vi "AIT 1553 - ReadWrite Message.vi"(5 "Mode":T9, 7 "Iteration":i32, 8 "error in (no error)":errorcluster, 9 "Bus Section":T1, 10 "FIFOs In":T2, 11 "Message In":T3 {"Driver Data"."First Word" min=8 max=31; "Driver Data"."Num Bits" min=1 max=32; "Driver Data"."Start Bit" min=8 max=31; "Block Data Refs"."Data Reference" format="%.0x"}) -> (0 "error out":errorcluster, 2 "FIFOs Out":T2, 3 "Message Out":T3 {"Driver Data"."First Word" min=8 max=31; "Driver Data"."Num Bits" min=1 max=32; "Driver Data"."Start Bit" min=8 max=31; "Block Data Refs"."Data Reference" format="%.0x"})   [LabVIEW 2014, in "AIT 1553 Custom Device.lvlib"]
uses:
  AIT 1553 Custom Device.lvlib
  RT Controls/ReadWrite Selector.ctl
  RT Controls/AIT 1553 - RT Message Settings.ctl
  <vilib>/NI Veristand/Custom Device API/Block Data Reference.ctl
  <vilib>/NI Veristand/Custom Device API/Data Reference.ctl
  RT Controls/AIT 1553 - Driver Data.ctl
  Controls and Global/Start Bit.ctl
  Controls and Global/Number of Bits.ctl
  RT Controls/FIFO.ctl
  RT Controls/AIT 1553 - Bus Section.ctl
  <vilib>/NI Veristand/Custom Device API/Global Data Refs.vi
  <vilib>/NI Veristand/Custom Device API/Custom Device API.lvlib
  <vilib>/NI Veristand/Custom Device Tools/Custom Device Utility Library/Custom Device Utility Library.lvlib
  <vilib>/NI Veristand/Custom Device Tools/Custom Device Utility Library/RT Debug String Color Spec.ctl
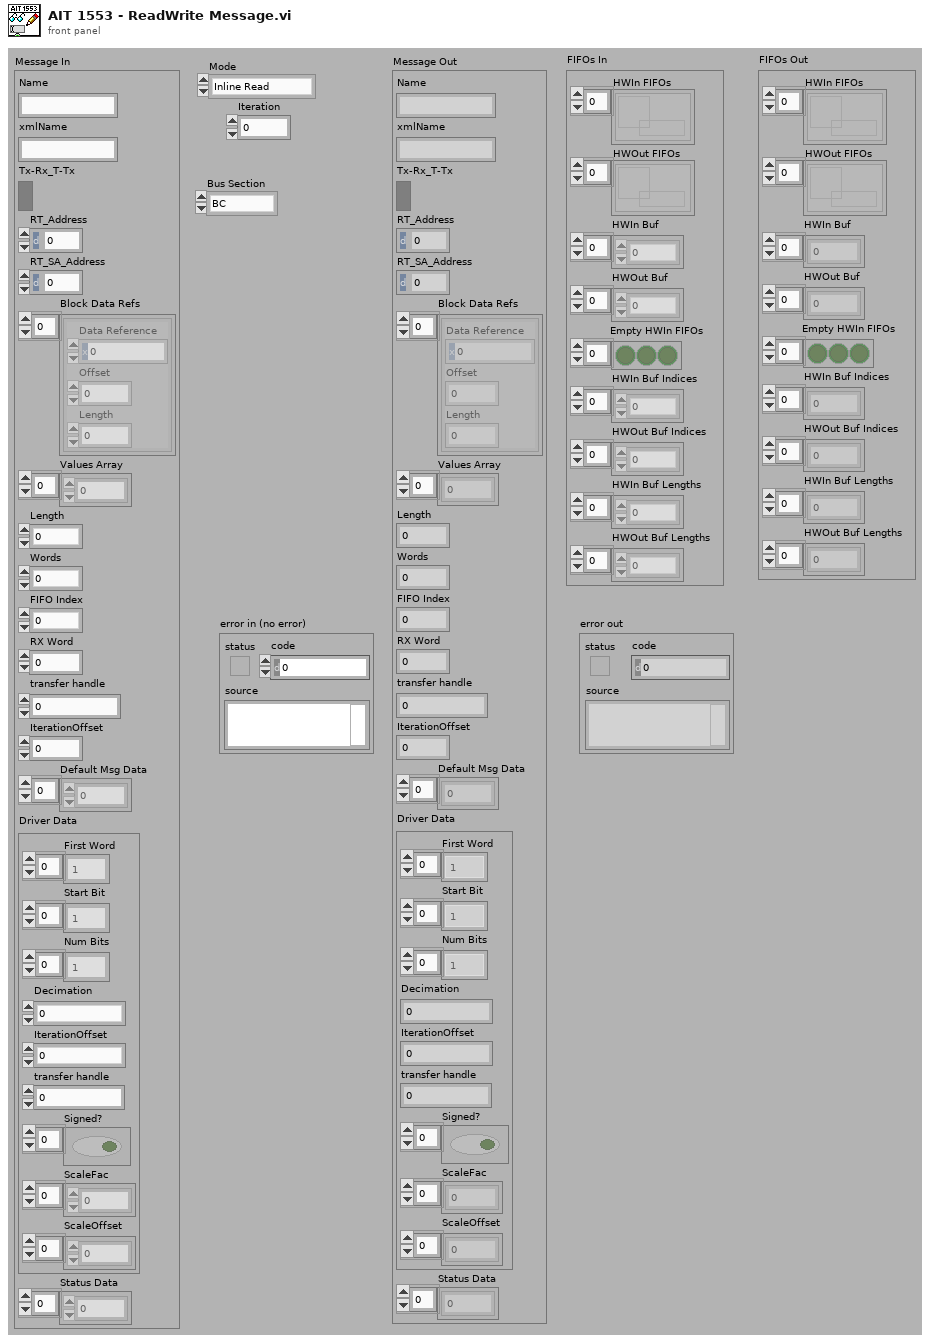
[diagram p1: front panel]
types:
  T1 = typedef "AIT 1553 Custom Device.lvlib/AIT 1553 - Bus Section.ctl" = enum16{"BC", "BM", "RT"}
  T2 = typedef "AIT 1553 Custom Device.lvlib/FIFO.ctl" = cluster{"HWIn FIFOs":refnum<k33>[], "HWOut FIFOs":refnum<k33>[], "HWIn Buf":dbl[], "HWOut Buf":dbl[], "Empty HWIn FIFOs":bool[], "HWIn Buf Indices":i32[], "HWOut Buf Indices":i32[], "HWIn Buf Lengths":i32[], "HWOut Buf Lengths":i32[]}
  T3 = typedef "AIT 1553 Custom Device.lvlib/AIT 1553 - RT Message Settings.ctl" = cluster{"Name":string, "xmlName":string, "Tx-Rx_T-Tx":bool, "RT_Address":u8, "RT_SA_Address":u8, "Block Data Refs":T4[], "Values Array":dbl[], "Length":i32, "Words":i32, "FIFO Index":i32, "RX Word":u32, "transfer handle":u32, "IterationOffset":i32, "Default Msg Data":u16[], "Driver Data":T6, "Status Data":u32[]}
  T4 = typedef "Custom Device API.lvlib/Block Data Reference.ctl" = cluster{"Data Reference":T5, "Offset":i32, "Length":i32}
  T5 = typedef "Custom Device API.lvlib/Data Reference.ctl" = i32
  T6 = typedef "AIT 1553 Custom Device.lvlib/AIT 1553 - Driver Data.ctl" = cluster{"First Word":T7[], "Start Bit":T7[], "Num Bits":T8[], "Decimation":i32, "IterationOffset":i32, "transfer handle":u32, "Signed?":bool[], "ScaleFac":dbl[], "ScaleOffset":dbl[]}
  T7 = typedef "AIT 1553 Custom Device.lvlib/Start Bit.ctl" = i32
  T8 = typedef "AIT 1553 Custom Device.lvlib/Number of Bits.ctl" = i32
  T9 = typedef "AIT 1553 Custom Device.lvlib/ReadWrite Selector.ctl" = enum16{"Inline Read", "Inline Write", "Async HWIn", "Async HWOut"}
  T10 = typedef "Custom Device Utility Library.lvlib/RT Debug String Color Spec.ctl" = u16
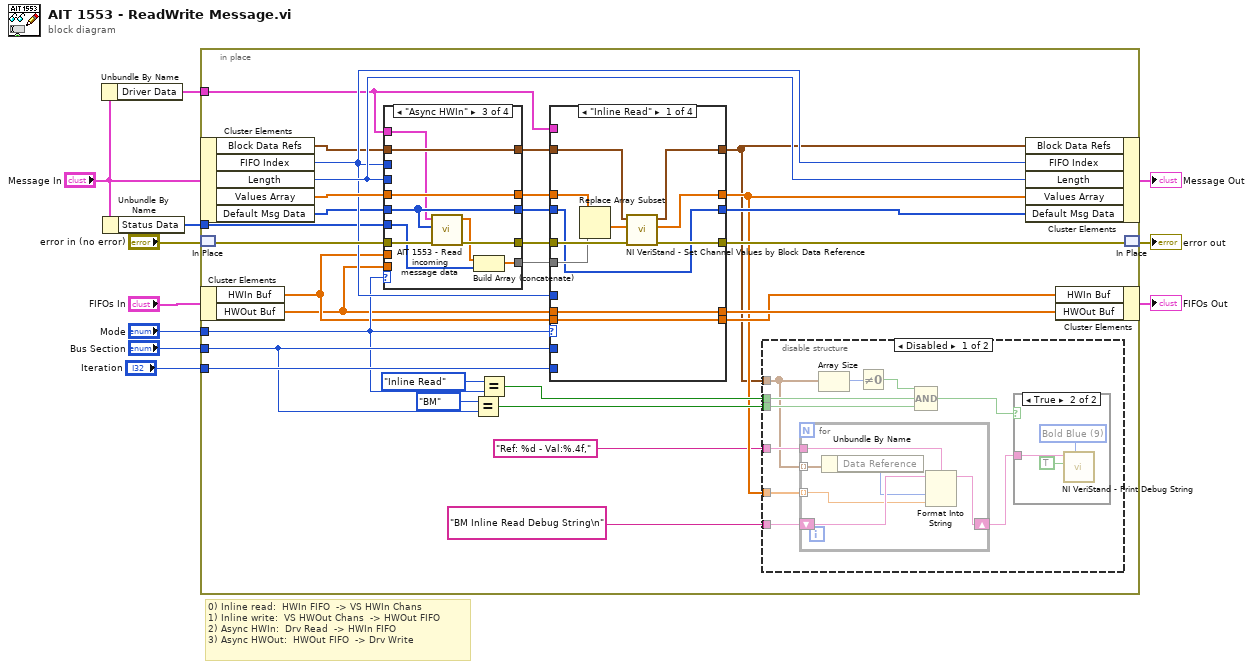
[diagram p0: block diagram]
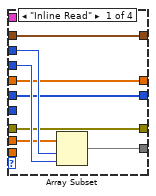
[diagram p4: hidden frame]
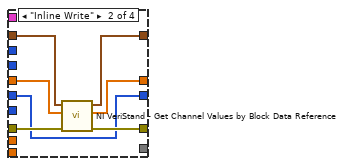
[diagram p5: hidden frame]
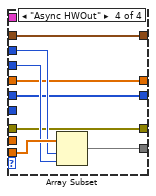
[diagram p6: hidden frame]
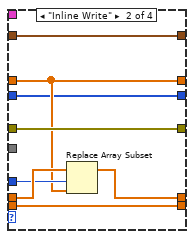
[diagram p7: hidden frame]
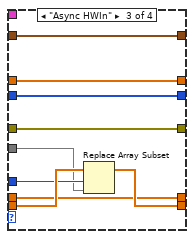
[diagram p8: hidden frame]
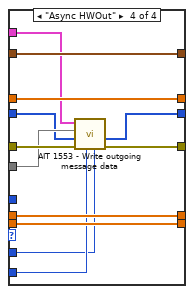
[diagram p9: hidden frame]
diagram:
  # "0) Inline read:\t\tHWIn FIFO \t-> VS HWIn Chans\n1) Inline write: \tVS HWOut Chans \t-> HWOut FIFO\n2) Async HWIn:\t\tDrv Read \t-> HWIn FIFO\n3) Async HWOut: \tHWOut FIFO \t-> Drv Write"
  n1 = Unbundle By Name("Message In") -> ("Driver Data"=w3:T6)
  n2 = Unbundle By Name("Message In") -> ("Status Data"=w1:u32[])
  n3 = in-place {
    in-place-border: "Mode" -> [w24]
    in-place-border: "Iteration" -> [w30]
    in-place-border: "Bus Section" -> [w26]
    in-place-border: w3 -> [w13]
    in-place-border: w1 -> [w12]
    n4 = in-place-cluster #1("Message In") -> ("Block Data Refs"=w17:T4[], "FIFO Index"=w32:i32, "Length"=w39:i32, "Values Array"=w36:dbl[], "Default Msg Data"=w29:u16[])
    n5 = in-place-match #2("error in (no error)") -> (w38:errorcluster)
    n6 = in-place-cluster #3("FIFOs In") -> ("HWIn Buf"=w15:dbl[], "HWOut Buf"=w14:dbl[])
    n7 = case shown="\"Async HWIn\"" w24 {
      tunnel: w15 -> [w65 _ _ _]
      tunnel: w32 -> [w68 _ _ w91]
      tunnel: w39 -> [w67 _ _ w90]
      tunnel: [w66 _ w77 w86] -> w41
      tunnel: w38 -> [w62 w75 w82 w87]
      tunnel: [w62 w74 w81 w87] -> w37
      tunnel: w17 -> [w64 w73 w84 w88]
      tunnel: w36 -> [w63 w72 w83 w89]
      tunnel: [w63 w71 w83 w89] -> w34
      tunnel: [w64 w70 w84 w88] -> w35
      tunnel: w13 -> [_ _ w79 _]
      tunnel: w14 -> [_ _ _ w92]
      tunnel: w29 -> [w61 w69 w80 w85]
      tunnel: [w61 w69 w80 w85] -> w28
      tunnel: w12 -> [_ _ w76 _]
      frame "Inline Read" {
        n8 = Array Subset(array=w65, index=w68, length=w67) -> (w66:dbl[])
      }
      frame "Inline Write" {
        n9 = call <vilib>:"NI VeriStand - Get Channel Values by Block Data Reference.vi"("error in (no error)"=w75, "Values Array in"=w72, "Block Data Ref"=w73) -> ("error out"=w74:errorcluster, "Values Array out"=w71:dbl[], "Block Data Ref dup"=w70:T4[])  [unwired: 6 in]
      }
      frame "Async HWIn" {
        n10 = call "AIT 1553 - Read incoming message data.vi"("error in (no error)"=w82, "Default Msg Data"=w80, "Driver Data"=w79) -> ("error out"=w81:errorcluster, "Values"=w78:dbl[])  [unwired: 7 in]
        n11 = Build Array (concatenate)(w78, w76) -> (w77:dbl[])
      }
      frame "Async HWOut" {
        n12 = Array Subset(array=w92, index=w91, length=w90) -> (w86:dbl[])
      }
    }
    n13 = Equal?(x=AIT_1553_-_Bus_Section."BM", y=w26) -> (x = y?=w22:bool)
    n14 = Equal?(x=ReadWrite_Selector."Inline Read", y=w24) -> (x = y?=w21:bool)
    n15 = case shown="\"Inline Read\"" w24 {
      tunnel: w35 -> [w96 w108 w120 w130]
      tunnel: w41 -> [w101 _ w113 w128]
      tunnel: w37 -> [w103 w109 w116 w129]
      tunnel: [w102 w109 w116 w127] -> w40
      tunnel: w34 -> [w95 w107 w114 w122]
      tunnel: [w100 w107 w114 w122] -> w20
      tunnel: [w99 w108 w120 w130] -> w16
      tunnel: w14 -> [w98 w111 w115 w131]
      tunnel: [w98 w104 w115 w131] -> w33
      tunnel: w32 -> [_ w110 w117 _]
      tunnel: w15 -> [w97 w106 w119 w132]
      tunnel: [w97 w106 w118 w132] -> w31
      tunnel: w13 -> [_ _ _ w121]
      tunnel: w30 -> [_ _ _ w126]
      tunnel: w28 -> [w93 w105 w112 w125]
      tunnel: [w93 w105 w112 w124] -> w27
      tunnel: w26 -> [_ _ _ w123]
      frame "Inline Read" {
        n16 = Replace Array Subset(array=w95, new element=w101) -> (w94:dbl[])  [unwired: 1 in]
        n17 = call <vilib>:"NI VeriStand - Set Channel Values by Block Data Reference.vi"("error in (no error)"=w103, "Values Array in"=w94, "Block Data Ref"=w96) -> ("error out"=w102:errorcluster, "Values Array out"=w100:dbl[], "Block Data Ref dup"=w99:T4[])  [unwired: 6 in]
      }
      frame "Inline Write" {
        n18 = Replace Array Subset(array=w111, new element=w107, index=w110) -> (w104:dbl[])
      }
      frame "Async HWIn" {
        n19 = Replace Array Subset(array=w119, new element=w113, index=w117) -> (w118:dbl[])
      }
      frame "Async HWOut" {
        n20 = call "AIT 1553 - Write outgoing message data.vi"("Bus Section"=w123, "Iteration"=w126, "error in (no error)"=w129, "Msg Data In"=w125, "Values"=w128, "Driver Data"=w121) -> ("error out"=w127:errorcluster, "Msg Data Out"=w124:u16[])  [unwired: 4 in]
      }
    }
    n21 = disable-structure shown="Disabled" {
      disable-tunnel: w22 -> [w51 _]
      disable-tunnel: w21 -> [w50 _]
      disable-tunnel: w20 -> [w49 _]
      disable-tunnel: "Ref: %d - Val:%.4f," ("format string") -> [w48 _]
      disable-tunnel: "BM Inline Read Debug String\n" ("format string") -> [w46 _]
      disable-tunnel: w16 -> [w45 _]
      frame Disabled {
        n22 = for {
          tunnel: w45 -> [w57] mode=indexing
          tunnel: w49 -> [w53] mode=indexing
          shift-right: [w55] -> w42
          shift-left: w46 -> [w56]
          tunnel: w48 -> [w52]
          n23 = Unbundle By Name(w57) -> ("Data Reference"=w54:T5)
          n24 = Format Into String(format string=w52, initial string=w56, w54, w53) -> (resulting string=w55:string)  [unwired: 1 in, 1 out]
        }
        n25 = Array Size(array=w45) -> (size(s)=w47:i32)
        n26 = Not Equal To 0?(x=w47) -> (x != 0?=w44:bool)
        n27 = Compound Arithmetic op=AND(w44, w50, w51) -> (w43:bool)
        n28 = case shown="True" w43 {
          tunnel: w42 -> [_ w58]
          frame False {
          }
          frame True {
            w60 = T10 9 items=["Plain White"=7, "Bold White"=15, "Bold Blue"=9, "Bold Green"=10, "Bold Red"=12] ("Attribute")
            n29 = call <vilib>:"NI VeriStand - Print Debug String.vi"("Attribute"=w60, "Add to log file? (T)"=TRUE, "Message"=w58) -> ()  [unwired: 8 in, 1 out]
          }
        }
      }
      frame Enabled {
      }
    }
    n30 = in-place-cluster #1("Block Data Refs"=w16, "FIFO Index"=w32, "Length"=w39, "Values Array"=w20, "Default Msg Data"=w27) -> (→"Message Out":T3)
    n31 = in-place-cluster #3("HWIn Buf"=w31, "HWOut Buf"=w33) -> (→"FIFOs Out":T2)
    n32 = in-place-match #2(w40) -> (→"error out":errorcluster)
  }
